vi "NIPKG Utility.vi"() -> ()   [LabVIEW 2017]
uses:
  <userlib>/_OpenG.lib/file/file.llb/Valid Path - Traditional__ogtk.vi
panel:
  out "State":string
  in  "Quit":bool
  in  "Tab Control":enum32{"Unpack NIPKG", "Pack NIPKG"}(tab)
  out "Unpack Complete?":bool
  out "Unpack Status":string
  in  "Unpack":bool
  in  "Path to .NIPKG":path
  in  "Unpack Destination":path
  in  "View Unpack Folder":bool
  in  "open":bool
  in  "Pack":bool
  in  "Path to Package Source":path
  in  "Pack Destination":path
  out "Pack Status":string
  in  "View Pack Folder":bool
  out "Pack Complete?":bool
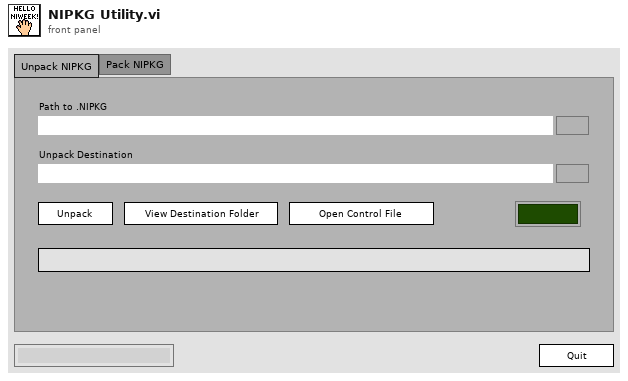
[diagram p1: front panel]
types:
  T1 = cluster{"unpack status":bool, "path to source":string, "pack destination":string, "pack status":string}
  T2 = cluster{"ready to unpack":bool, "path to nipkg":string, "unpack destination":string, "unpack status":string}
  T3 = cluster{"Core":cluster{"Current VI Reference":refnum<vi>, "Close Panel on Exit?":bool}, "unpack data":cluster{"ready to unpack":bool, "path to nipkg":string, "unpack destination":string, "unpack status":string}, "pack data":cluster{"ready to pack":bool, "path to source":string, "pack destination":string, "pack status":string}, "control path":string, "Unpack complete?":bool, "Pack complete?":bool}
  T4 = cluster{"ready to pack":bool, "path to source":string, "pack destination":string, "pack status":string}
  T5 = cluster{"Current VI Reference":refnum<vi>, "Close Panel on Exit?":bool}
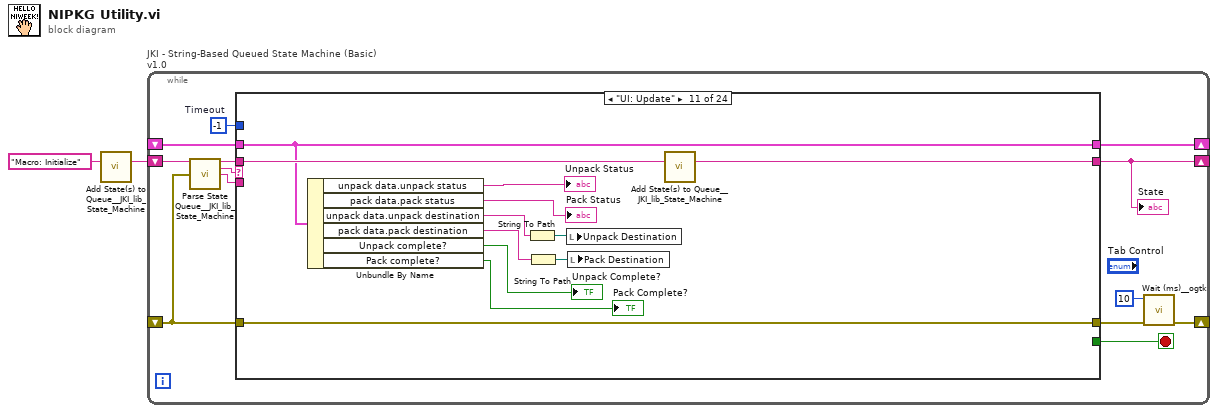
[diagram p0: block diagram]
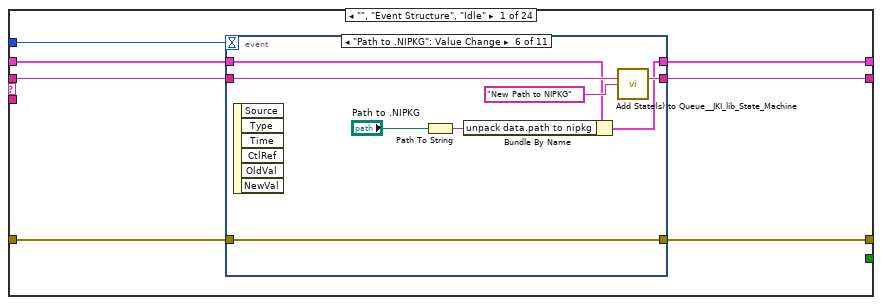
[diagram p2: hidden frame]
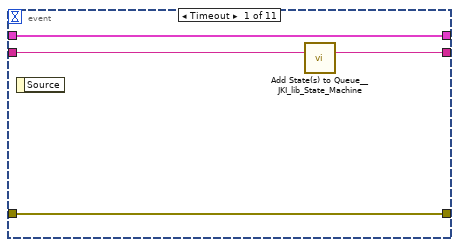
[diagram p3: hidden frame]
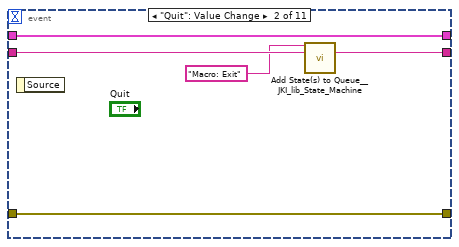
[diagram p4: hidden frame]
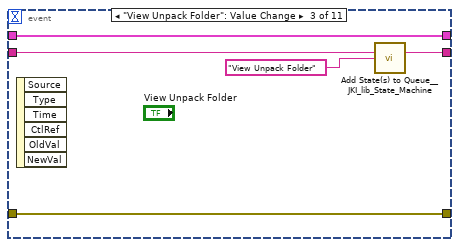
[diagram p5: hidden frame]
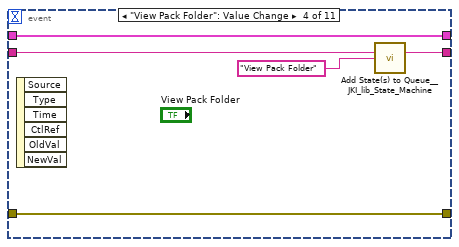
[diagram p6: hidden frame]
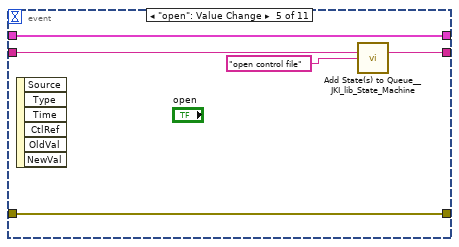
[diagram p7: hidden frame]
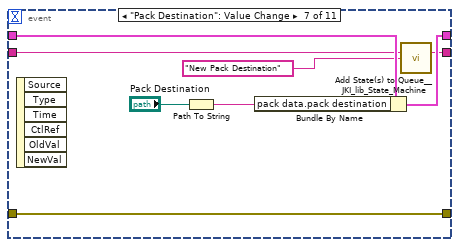
[diagram p8: hidden frame]
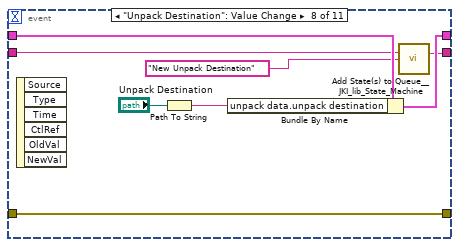
[diagram p9: hidden frame]
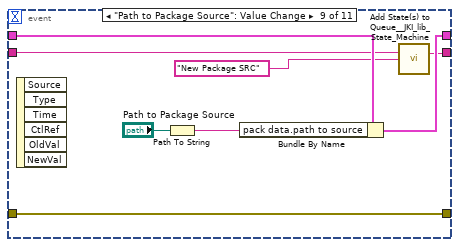
[diagram p10: hidden frame]
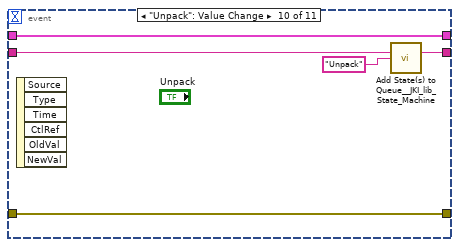
[diagram p11: hidden frame]
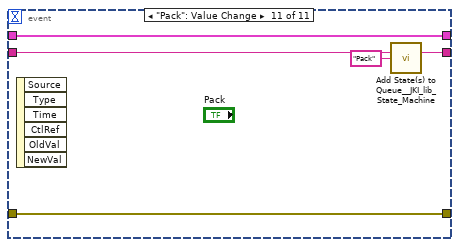
[diagram p12: hidden frame]
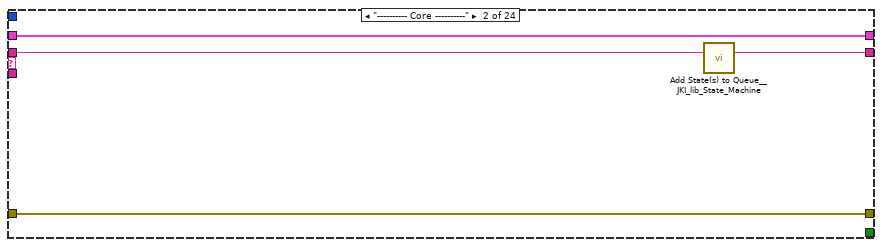
[diagram p13: hidden frame]
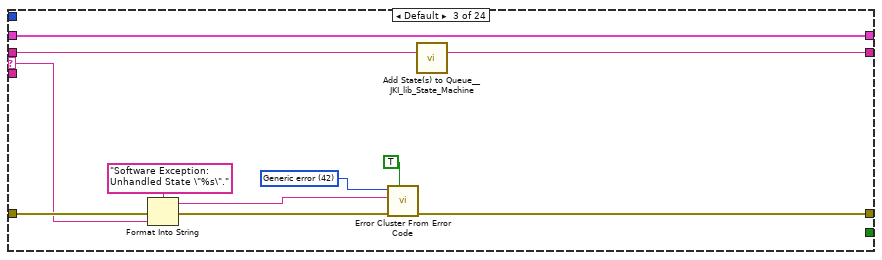
[diagram p14: hidden frame]
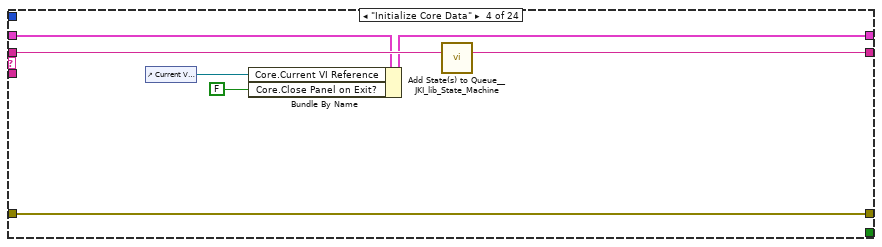
[diagram p15: hidden frame]
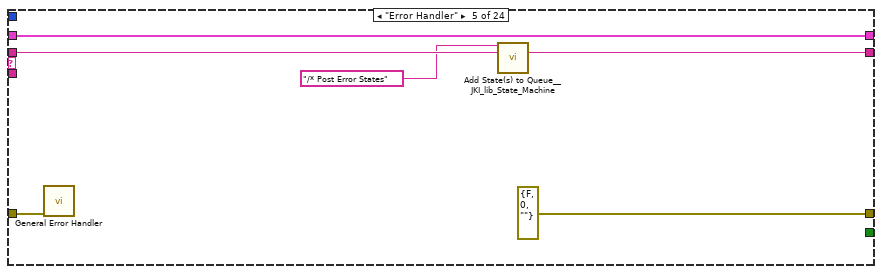
[diagram p16: hidden frame]
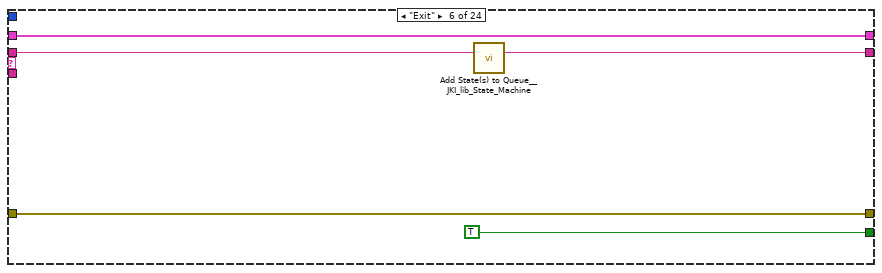
[diagram p17: hidden frame]
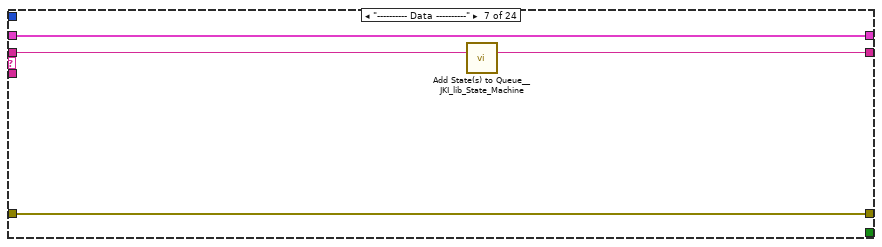
[diagram p18: hidden frame]
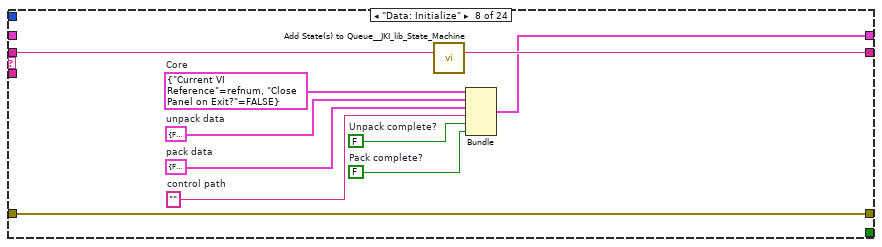
[diagram p19: hidden frame]
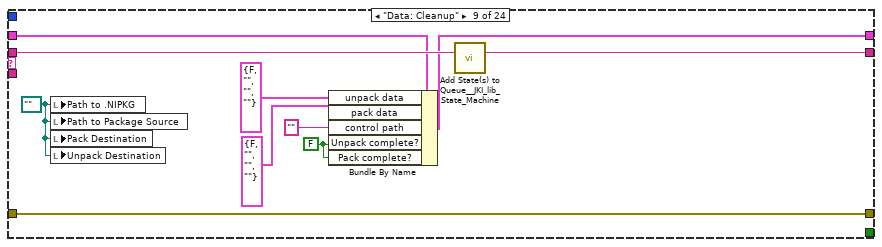
[diagram p20: hidden frame]
diagram:
  n1 = call <vilib>:"Add State(s) to Queue__JKI_lib_State_Machine.vi"("State(s) in (\"\")"="Macro: Initialize") -> ("States Out"=w1:string)  [unwired: 14 in]
  n2 = while "JKI - String-Based Queued State Machine (Basic) v1.0" {
    shift-right: [w10] -> _
    shift-left: _ -> [w9]
    shift-right: [w4] -> _
    shift-left: _ -> [w7]
    shift-right: [w6] -> _
    shift-left: w1 -> [w12]
    stop <- w11 stop-if-true
    w8 = -1  # Timeout
    n3 = call <vilib>:"Parse State Queue__JKI_lib_State_Machine.vi"("State Queue"=w12, "Error In (no error)"=w7) -> ("Remaining States"=w14:string, "Current State"=w15:string, "Arguments"=w13:string)  [unwired: 11 in]
    n4 = case shown="\"UI: Update\"" w15 {
      selector: w15 -> [_ _ w93 _ _ _ _ _ _ _ _ _ _ _ _ _ _ _ _ _ _ _ _ _]
      tunnel: w14 -> [w22 w92 w97 w110 w116 w121 w125 w135 w145 w149 w161 w165 w170 w177 w181 w198 w216 w224 w239 w256 w274 w296 w314 w329]
      tunnel: w13 -> [_ _ _ _ _ _ _ _ _ _ _ _ _ _ _ _ _ _ _ _ _ _ _ _]
      tunnel: w9 -> [w20 w89 w95 w106 w113 w119 w122 _ w142 w146 w158 w162 w167 w174 w178 w189 w207 w222 w237 w251 w269 w291 w309 w324]
      tunnel: [w19 w90 w99 w107 errorcluster {"status"=FALSE, "code"=0, "source"=""} ("error out") w118 w123 w132 w143 w147 w159 w163 w168 w175 w179 w195 w213 w220 w236 w253 w272 w294 w312 w327] -> w5
      tunnel: w7 -> [w18 w90 w98 w107 w112 w118 w123 w132 w143 w147 w159 w163 w168 w175 w179 w196 w214 w221 w235 w254 w272 w294 w312 w327]
      tunnel: [w21 w91 w96 w109 w115 w120 w124 w134 w144 w148 w160 w164 w169 w176 w180 w197 w215 w223 w238 w255 w273 w295 w313 w328] -> w6
      tunnel: [_ _ _ _ _ TRUE _ _ _ _ _ _ _ _ _ _ _ _ _ _ _ _ _ _] -> w11
      tunnel: [w17 w89 w95 w108 w113 w119 w122 w133 w141 w146 w158 w162 w167 w174 w178 w188 w206 w222 w237 w251 w270 w292 w310 w325] -> w10
      tunnel: w8 -> [w16 _ _ _ _ _ _ _ _ _ _ _ _ _ _ _ _ _ _ _ _ _ _ _]
      frame "", "Event Structure", "Idle" {
        n5 = event shown="[5] \"Path to .NIPKG\": Value Change" {
          selector: _ -> [_ _ _ _ _ _ _ _ _ _ _]
          dyn-events: _ -> [_ _ _ _ _ _ _ _ _ _ _]
          timeout: w16 -> [_ _ _ _ _ _ _ _ _ _ _]
          tunnel: w22 -> [w26 w31 w35 w40 w45 w53 w58 w66 w74 w82 w87]
          tunnel: [w25 w30 w36 w41 w46 w54 w60 w67 w75 w83 w88] -> w21
          tunnel: w20 -> [w23 w28 w34 w39 w42 w48 w61 w69 w77 w80 w85]
          tunnel: [w24 w29 w33 w38 w44 w51 w55 w63 w71 w81 w86] -> w19
          tunnel: w18 -> [w24 w29 w33 w38 w44 w51 w55 w63 w71 w81 w86]
          tunnel: [w23 w28 w34 w39 w42 w47 w62 w68 w76 w80 w85] -> w17
          event Timeout {
            n6 = event-data() -> ()  [unwired: 1 in, 1 out]
            n7 = call <vilib>:"Add State(s) to Queue__JKI_lib_State_Machine.vi"("State(s) in (\"\")"=w26) -> ("States Out"=w25:string)  [unwired: 14 in]
          }
          event "Quit": Value Change {
            n8 = event-data() -> ()  [unwired: 1 in, 1 out]
            n9 = call <vilib>:"Add State(s) to Queue__JKI_lib_State_Machine.vi"("State(s) in Front (\"\")"="Macro: Exit", "State(s) in (\"\")"=w31) -> ("States Out"=w30:string)  [unwired: 13 in]
          }
          event "View Unpack Folder": Value Change {
            n10 = event-data() -> ()  [unwired: 1 in, 6 out]
            n11 = call <vilib>:"Add State(s) to Queue__JKI_lib_State_Machine.vi"("State(s) in (\"\")"=w35, "State(s) at Back (\"\")"="View Unpack Folder" ("State(s) at Back (\"\")")) -> ("States Out"=w36:string)  [unwired: 13 in]
          }
          event "View Pack Folder": Value Change {
            n12 = event-data() -> ()  [unwired: 1 in, 6 out]
            n13 = call <vilib>:"Add State(s) to Queue__JKI_lib_State_Machine.vi"("State(s) in (\"\")"=w40, "State(s) at Back (\"\")"="View Pack Folder" ("State(s) at Back (\"\")")) -> ("States Out"=w41:string)  [unwired: 13 in]
          }
          event "open": Value Change {
            n14 = event-data() -> ()  [unwired: 1 in, 6 out]
            n15 = call <vilib>:"Add State(s) to Queue__JKI_lib_State_Machine.vi"("State(s) in (\"\")"=w45, "State(s) at Back (\"\")"="open control file") -> ("States Out"=w46:string)  [unwired: 13 in]
          }
          event "Path to .NIPKG": Value Change {
            n16 = event-data() -> ()  [unwired: 1 in, 6 out]
            n17 = Path To String(path="Path to .NIPKG") -> (string=w49:string)
            n18 = Bundle By Name(cluster=w48, "unpack data.path to nipkg"=w49) -> (w47:T3)
            n19 = call <vilib>:"Add State(s) to Queue__JKI_lib_State_Machine.vi"("State(s) in (\"\")"=w53, "State(s) at Back (\"\")"="New Path to NIPKG" ("State(s) at Back (\"\")")) -> ("States Out"=w54:string)  [unwired: 13 in]
          }
          event "Pack Destination": Value Change {
            n20 = event-data() -> ()  [unwired: 1 in, 6 out]
            n21 = Path To String(path="Pack Destination") -> (string=w59:string)
            n22 = Bundle By Name(cluster=w61, "pack data.pack destination"=w59) -> (w62:T3)
            n23 = call <vilib>:"Add State(s) to Queue__JKI_lib_State_Machine.vi"("State(s) in (\"\")"=w58, "State(s) at Back (\"\")"="New Pack Destination" ("State(s) at Back (\"\")")) -> ("States Out"=w60:string)  [unwired: 13 in]
          }
          event "Unpack Destination": Value Change {
            n24 = event-data() -> ()  [unwired: 1 in, 6 out]
            n25 = Path To String(path="Unpack Destination") -> (string=w70:string)
            n26 = Bundle By Name(cluster=w69, "unpack data.unpack destination"=w70) -> (w68:T3)
            n27 = call <vilib>:"Add State(s) to Queue__JKI_lib_State_Machine.vi"("State(s) in (\"\")"=w66, "State(s) at Back (\"\")"="New Unpack Destination" ("State(s) at Back (\"\")")) -> ("States Out"=w67:string)  [unwired: 13 in]
          }
          event "Path to Package Source": Value Change {
            n28 = event-data() -> ()  [unwired: 1 in, 6 out]
            n29 = Path To String(path="Path to Package Source") -> (string=w78:string)
            n30 = Bundle By Name(cluster=w77, "pack data.path to source"=w78) -> (w76:T3)
            n31 = call <vilib>:"Add State(s) to Queue__JKI_lib_State_Machine.vi"("State(s) in (\"\")"=w74, "State(s) at Back (\"\")"="New Package SRC" ("State(s) at Back (\"\")")) -> ("States Out"=w75:string)  [unwired: 13 in]
          }
          event "Unpack": Value Change {
            n32 = event-data() -> ()  [unwired: 1 in, 6 out]
            n33 = call <vilib>:"Add State(s) to Queue__JKI_lib_State_Machine.vi"("State(s) in (\"\")"=w82, "State(s) at Back (\"\")"="Unpack" ("State(s) at Back (\"\")")) -> ("States Out"=w83:string)  [unwired: 13 in]
          }
          event "Pack": Value Change {
            n34 = event-data() -> ()  [unwired: 1 in, 6 out]
            n35 = call <vilib>:"Add State(s) to Queue__JKI_lib_State_Machine.vi"("State(s) in (\"\")"=w87, "State(s) at Back (\"\")"="Pack" ("State(s) at Back (\"\")")) -> ("States Out"=w88:string)  [unwired: 13 in]
          }
        }
      }
      frame "---------- Core ----------" {
        n36 = call <vilib>:"Add State(s) to Queue__JKI_lib_State_Machine.vi"("State(s) in (\"\")"=w92) -> ("States Out"=w91:string)  [unwired: 14 in]
      }
      frame Default {
        w102 = 42 items=["No error", "Argument error", "Memory is full", "Out of zone", "End of file", "File already open", "Generic file I/O error", "File not found", "File permission error", "Disk is full", "Duplicate path", "Too many files open", "System feature not enabled", "Resource file not found", "Cannot add resource", "Resource not found", "Image not found", "Image memory error", "Pen does not exist", "Config type invalid", "Config token not found", "Config parse error", "Config memory error", "Bad external code format", "Bad external code offset", "External code not present", "Null window", "Destroy window error", "Null menu", "Print aborted", "Bad print record", "Print driver error", "Windows error during printing", "Memory error during printing", "Print dialog error", "Generic print error", "Invalid device refnum", "Device not found", "Device parameter error", "Device unit error", "Cannot open device", "Device call aborted", "Generic error", "Cancelled by user", "Object ID too low", "Object ID too high", "Object not in heap", "Unknown heap", "Unknown object (invalid DefProc)", "Unknown object (DefProc not in table)", "Message out of range", "Invalid (null) method", "Unknown message", "Manager call not supported", "Bad address", "Network operation in progress", "Network operation timed out", "Connection is busy", "Network attribute not supported", "Network error", "Address in use", "System out of memory", "Connection aborted", "Connection refused", "Not connected", "Already connected", "Connection closed", "Initialization error (interapplication manager)", "Bad occurrence", "Wait on unbound occurrence handler", "Occurrence queue overflow", "Datalog type conflict", "Unused", "Unrecognized type (interapplication manager)", "Memory corrupt", "Failed to make temporary DLL", "Old CIN version", "Drag socket not found", "Failed to load drop-object", "Failed to register OLE object", "Failed to release OLE object", "Format specifier type mismatch", "Unknown format specifier", "Too few format specifiers", "Too many format specifiers", "Scan failed", "Newer CIN version", "Error converting to variant", "Runtime menu error", "Password tampered", "Variant attribute not found", "Incompatible variant data type", "Event data is not available", "Event Store is not present", "Occurrence is not found", "Event Queue is not created", "Event info is not available", "Refnum passed is NULL", "Error retrieving Class GUID", "Error retrieving CoClass GUID", "Error retrieving TypeLib GUID.", "Bad built application magic bytes.", "Specific driver is different from the specific driver associated with the Logical Name.", "There is no session opened to the class driver.", "Max Error", "MAX - Error with config objects", "MAX - Error loading configuration", "MAX - Group not supported"]
        n37 = Format Into String(format string="Software Exception: Unhandled State \"%s\"." ("message"), error in=w98, w93) -> (resulting string=w101:string, error out=w100:errorcluster)  [unwired: 1 in]
        n38 = call <vilib>:"Error Cluster From Error Code.vi"("show call chain? (False)"=TRUE, "error in (no error)"=w100, "error message (\"\")"=w101, "error code (0)"=w102) -> ("error out"=w99:errorcluster)  [unwired: 5 in]
        n39 = call <vilib>:"Add State(s) to Queue__JKI_lib_State_Machine.vi"("State(s) in (\"\")"=w97) -> ("States Out"=w96:string)  [unwired: 14 in]
      }
      frame "Initialize Core Data" {
        n40 = control-ref of="Current VI Reference"() -> (w105:refnum<vi>)
        n41 = Bundle By Name(cluster=w106, "Core.Current VI Reference"=w105, "Core.Close Panel on Exit?"=FALSE) -> (w108:T3)
        n42 = call <vilib>:"Add State(s) to Queue__JKI_lib_State_Machine.vi"("State(s) in (\"\")"=w110) -> ("States Out"=w109:string)  [unwired: 14 in]
      }
      frame "Error Handler" {
        n43 = call <vilib>:"General Error Handler.vi"("error in (no error)"=w112) -> ()  [unwired: 10 in, 5 out]
        n44 = call <vilib>:"Add State(s) to Queue__JKI_lib_State_Machine.vi"("State(s) in Front (\"\")"="/* Post Error States", "State(s) in (\"\")"=w116) -> ("States Out"=w115:string)  [unwired: 13 in]
      }
      frame "Exit" {
        n45 = call <vilib>:"Add State(s) to Queue__JKI_lib_State_Machine.vi"("State(s) in (\"\")"=w121) -> ("States Out"=w120:string)  [unwired: 14 in]
      }
      frame "---------- Data ----------" {
        n46 = call <vilib>:"Add State(s) to Queue__JKI_lib_State_Machine.vi"("State(s) in (\"\")"=w125) -> ("States Out"=w124:string)  [unwired: 14 in]
      }
      frame "Data: Initialize" {
        w126 = FALSE  # Pack complete?
        w127 = FALSE  # Unpack complete?
        w128 = ""  # control path
        w129 = T4 {"ready to pack"=FALSE, "path to source"="", "pack destination"="", "pack status"="Please specify the path to the ni package source folder..."}  # pack data
        w130 = T2 {"ready to unpack"=FALSE, "path to nipkg"="", "unpack destination"="", "unpack status"="Please specify the path to an NI package file..."}  # unpack data
        w131 = T5 {"Current VI Reference"=refnum, "Close Panel on Exit?"=FALSE}  # Core
        n47 = call <vilib>:"Add State(s) to Queue__JKI_lib_State_Machine.vi"("State(s) in (\"\")"=w135) -> ("States Out"=w134:string)  [unwired: 14 in]
        n48 = Bundle("Core"=w131, "unpack data"=w130, "pack data"=w129, "control path"=w128, "Unpack complete?"=w127, "Pack complete?"=w126) -> (w133:T3)  [unwired: 1 in]
      }
      frame "Data: Cleanup" {
        w136 = FALSE
        w137 = path "" ("Path to .NIPKG")
        n49 = local write "Path to .NIPKG"(w137) -> ()
        n50 = local write "Path to Package Source"(w137) -> ()
        n51 = local write "Pack Destination"(w137) -> ()
        n52 = local write "Unpack Destination"(w137) -> ()
        n53 = Bundle By Name(cluster=w142, "unpack data"=T2 {"ready to unpack"=FALSE, "path to nipkg"="", "unpack destination"="", "unpack status"=""}, "pack data"=T1 {"unpack status"=FALSE, "path to source"="", "pack destination"="", "pack status"=""}, "control path"="", "Unpack complete?"=w136, "Pack complete?"=w136) -> (w141:T3)
        n54 = call <vilib>:"Add State(s) to Queue__JKI_lib_State_Machine.vi"("State(s) in (\"\")"=w145) -> ("States Out"=w144:string)  [unwired: 14 in]
      }
      frame "---------- UI ----------" {
        n55 = call <vilib>:"Add State(s) to Queue__JKI_lib_State_Machine.vi"("State(s) in (\"\")"=w149) -> ("States Out"=w148:string)  [unwired: 14 in]
      }
      frame "UI: Update" {
        n56 = Unbundle By Name(w158) -> ("unpack data.unpack status"=→"Unpack Status":string, "pack data.pack status"=→"Pack Status":string, "unpack data.unpack destination"=w153:string, "pack data.pack destination"=w152:string, "Unpack complete?"=→"Unpack Complete?":bool, "Pack complete?"=→"Pack Complete?":bool)
        n57 = String To Path(string=w153) -> (path=w155:path)
        n58 = String To Path(string=w152) -> (path=w154:path)
        n59 = local write "Unpack Destination"(w155) -> ()
        n60 = local write "Pack Destination"(w154) -> ()
        n61 = call <vilib>:"Add State(s) to Queue__JKI_lib_State_Machine.vi"("State(s) in (\"\")"=w161) -> ("States Out"=w160:string)  [unwired: 14 in]
      }
      frame "---------- Macro ----------" {
        n62 = call <vilib>:"Add State(s) to Queue__JKI_lib_State_Machine.vi"("State(s) in (\"\")"=w165) -> ("States Out"=w164:string)  [unwired: 14 in]
      }
      frame "Macro: Initialize" {
        n63 = call <vilib>:"Add State(s) to Queue__JKI_lib_State_Machine.vi"("State(s) in Front (\"\")"="Data: Initialize\nInitialize Core Data\nUI: Update", "State(s) in (\"\")"=w170) -> ("States Out"=w169:string)  [unwired: 13 in]
      }
      frame "Macro: Exit" {
        n64 = call <vilib>:"Add State(s) to Queue__JKI_lib_State_Machine.vi"("State(s) in (\"\")"="", "State(s) at Back (\"\")"="Data: Cleanup\nUI: Update\nExit") -> ("States Out"=w172:string)  [unwired: 13 in]
        n65 = call <vilib>:"Add State(s) to Queue__JKI_lib_State_Machine.vi"("State(s) in Front (\"\")"=w172, "State(s) in (\"\")"=w177) -> ("States Out"=w176:string)  [unwired: 13 in]
      }
      frame "---------- New Category ----------" {
        n66 = call <vilib>:"Add State(s) to Queue__JKI_lib_State_Machine.vi"("State(s) in (\"\")"=w181) -> ("States Out"=w180:string)  [unwired: 14 in]
      }
      frame "Unpack" {
        w190 = "\""
        n67 = Unbundle By Name(w189) -> ("unpack data.path to nipkg"=w192:string, "unpack data.unpack destination"=w191:string)
        n68 = call <vilib>:"Space Constant.vi"() -> ("String"=w186:string)
        n69 = Concatenate Strings("cmd /c nipkg.exe", w186, "unpack", w186, w190, w192, w190, w186, w190, w191, w190) -> (w184:string)
        n70 = call <vilib>:"Add State(s) to Queue__JKI_lib_State_Machine.vi"("State(s) in (\"\")"=w198, "State(s) at Back (\"\")"="View Unpack Folder\nUI: Update" ("State(s) at Back (\"\")")) -> ("States Out"=w197:string)  [unwired: 13 in]
        n71 = call <vilib>:"System Exec.vi"("error in (no error)"=w196, "working directory"=path "c:/program files/national instruments/ni package manager", "command line"=w184) -> ("error out"=w195:errorcluster)  [unwired: 5 in, 3 out]
        n72 = Bundle By Name(cluster=w189, "unpack data.unpack status"="Unpacking complete!" ("string"), "Unpack complete?"=TRUE) -> (w188:T3)
      }
      frame "Pack" {
        w208 = "\""
        n73 = Unbundle By Name(w207) -> ("pack data.path to source"=w210:string, "pack data.pack destination"=w209:string)
        n74 = call <vilib>:"Space Constant.vi"() -> ("String"=w204:string)
        n75 = Concatenate Strings("cmd /c nipkg.exe", w204, "pack", w204, w208, w210, w208, w204, w208, w209, w208) -> (w202:string)
        n76 = call <vilib>:"Add State(s) to Queue__JKI_lib_State_Machine.vi"("State(s) in (\"\")"=w216, "State(s) at Back (\"\")"="View Pack Folder\nUI: Update" ("State(s) at Back (\"\")")) -> ("States Out"=w215:string)  [unwired: 13 in]
        n77 = call <vilib>:"System Exec.vi"("error in (no error)"=w214, "working directory"=path "c:/program files/national instruments/ni package manager", "command line"=w202) -> ("error out"=w213:errorcluster)  [unwired: 5 in, 3 out]
        n78 = Bundle By Name(cluster=w207, "pack data.pack status"="Packing complete!" ("string"), "pack data.ready to pack"=FALSE, "Pack complete?"=TRUE) -> (w206:T3)
      }
      frame "View Unpack Folder" {
        n79 = Unbundle By Name(w222) -> ("unpack data.unpack destination"=w218:string)
        n80 = String To Path(string=w218) -> (path=w219:path)
        n81 = call-poly <userlib>:"Valid Path__ogtk.vi"("path"=w219) -> ("valid"=w217:bool)
        n82 = case shown="True" w217 {
          tunnel: w221 -> [w225 w231]
          tunnel: [w225 w230] -> w220
          tunnel: w218 -> [_ w226]
          frame False {
          }
          frame True {
            n83 = Concatenate Strings("explorer.exe /select,\"", w226, "\"" ("string")) -> (w227:string)
            n84 = call <vilib>:"System Exec.vi"("error in (no error)"=w231, "command line"=w227) -> ("error out"=w230:errorcluster)  [unwired: 6 in, 3 out]
          }
        }
        n85 = call <vilib>:"Add State(s) to Queue__JKI_lib_State_Machine.vi"("State(s) in (\"\")"=w224) -> ("States Out"=w223:string)  [unwired: 14 in]
      }
      frame "View Pack Folder" {
        n86 = Unbundle By Name(w237) -> ("pack data.pack destination"=w233:string)
        n87 = String To Path(string=w233) -> (path=w234:path)
        n88 = call-poly <userlib>:"Valid Path__ogtk.vi"("path"=w234) -> ("valid"=w232:bool)
        n89 = case shown="True" w232 {
          tunnel: [w240 w243] -> w236
          tunnel: w235 -> [w240 w242]
          tunnel: w233 -> [_ w241]
          frame False {
          }
          frame True {
            n90 = Concatenate Strings("explorer.exe /select,\"", w241, "\"" ("string")) -> (w244:string)
            n91 = call <vilib>:"System Exec.vi"("error in (no error)"=w242, "command line"=w244) -> ("error out"=w243:errorcluster)  [unwired: 6 in, 3 out]
          }
        }
        n92 = call <vilib>:"Add State(s) to Queue__JKI_lib_State_Machine.vi"("State(s) in (\"\")"=w239) -> ("States Out"=w238:string)  [unwired: 14 in]
      }
      frame "open control file" {
        n93 = Unbundle By Name(w251) -> ("unpack data.unpack destination"=w250:string)
        n94 = Concatenate Strings(w250, "\\control" ("string")) -> (w249:string)
        n95 = String To Path(string=w249) -> (path=w248:path)
        n96 = call-poly <userlib>:"Valid Path__ogtk.vi"("path"=w248) -> ("valid"=w247:bool)
        n97 = case shown="True" w247 {
          tunnel: w254 -> [w257 w261]
          tunnel: [w257 w260] -> w253
          tunnel: w248 -> [_ w258]
          frame False {
          }
          frame True {
            n98 = call <vilib>:"System Exec.vi"("error in (no error)"=w261, "working directory"=w258, "command line"="cmd /c start notepad control") -> ("error out"=w260:errorcluster)  [unwired: 5 in, 3 out]
          }
        }
        n99 = call <vilib>:"Add State(s) to Queue__JKI_lib_State_Machine.vi"("State(s) in (\"\")"=w256) -> ("States Out"=w255:string)  [unwired: 14 in]
      }
      frame "New Path to NIPKG" {
        n100 = Unbundle By Name(w269) -> ("unpack data.path to nipkg"=w267:string)
        n101 = String To Path(string=w267) -> (path=w266:path)
        n102 = call-poly <userlib>:"Valid Path__ogtk.vi"("path"=w266) -> ("valid"=w268:bool)
        n103 = case shown="True" w268 {
          tunnel: w266 -> [_ w283]
          tunnel: [path "" ("appended path") w280] -> w265
          tunnel: [FALSE TRUE] -> w263
          tunnel: ["Please enter a valid path to the package file..." ("f") "Ready to unpack..." ("t")] -> w262
          frame False {
          }
          frame True {
            n104 = Strip Path(path=w283) -> (stripped path=w282:path)  [unwired: 1 out]
            n105 = Build Path(base path=w282, name or relative path="pkgsrc") -> (appended path=w280:path)
          }
        }
        n106 = Path To String(path=w265) -> (string=w264:string)
        n107 = Bundle By Name(cluster=w269, "unpack data.unpack destination"=w264, "unpack data.ready to unpack"=w263, "unpack data.unpack status"=w262) -> (w270:T3)
        n108 = call <vilib>:"Add State(s) to Queue__JKI_lib_State_Machine.vi"("State(s) in (\"\")"=w274, "State(s) at Back (\"\")"="UI: Update" ("State(s) at Back (\"\")")) -> ("States Out"=w273:string)  [unwired: 13 in]
      }
      frame "New Package SRC" {
        n109 = Unbundle By Name(w291) -> ("pack data.path to source"=w289:string)
        n110 = String To Path(string=w289) -> (path=w288:path)
        n111 = call-poly <userlib>:"Valid Path__ogtk.vi"("path"=w288) -> ("valid"=w290:bool)
        n112 = case shown="False" w290 {
          tunnel: w288 -> [_ w303]
          tunnel: [path "" ("appended path") w300] -> w287
          tunnel: [FALSE TRUE] -> w285
          tunnel: ["Please enter a valid path to the source..." ("f") "Ready to pack..." ("t")] -> w284
          frame False {
          }
          frame True {
            n113 = Strip Path(path=w303) -> (stripped path=w300:path)  [unwired: 1 out]
          }
        }
        n114 = Path To String(path=w287) -> (string=w286:string)
        n115 = Bundle By Name(cluster=w291, "pack data.pack destination"=w286, "pack data.ready to pack"=w285, "pack data.pack status"=w284) -> (w292:T3)
        n116 = call <vilib>:"Add State(s) to Queue__JKI_lib_State_Machine.vi"("State(s) in (\"\")"=w296, "State(s) at Back (\"\")"="UI: Update" ("State(s) at Back (\"\")")) -> ("States Out"=w295:string)  [unwired: 13 in]
      }
      frame "New Pack Destination" {
        n117 = Unbundle By Name(w309) -> ("pack data.pack destination"=w304:string)
        n118 = String To Path(string=w304) -> (path=w307:path)
        n119 = call-poly <userlib>:"Valid Path__ogtk.vi"("path"=w307) -> ("valid"=w308:bool)
        n120 = case shown="False" w308 {
          tunnel: [FALSE TRUE] -> w306
          tunnel: ["Please enter a valid destination path..." ("f") "Ready to unpack..." ("t")] -> w305
          frame False {
          }
          frame True {
          }
        }
        n121 = Bundle By Name(cluster=w309, "pack data.ready to pack"=w306, "pack data.pack destination"=w305) -> (w310:T3)
        n122 = call <vilib>:"Add State(s) to Queue__JKI_lib_State_Machine.vi"("State(s) in (\"\")"=w314, "State(s) at Back (\"\")"="UI: Update" ("State(s) at Back (\"\")")) -> ("States Out"=w313:string)  [unwired: 13 in]
      }
      frame "New Unpack Destination" {
        n123 = Unbundle By Name(w324) -> ("unpack data.unpack destination"=w319:string)
        n124 = String To Path(string=w319) -> (path=w322:path)
        n125 = call-poly <userlib>:"Valid Path__ogtk.vi"("path"=w322) -> ("valid"=w323:bool)
        n126 = case shown="False" w323 {
          tunnel: [FALSE TRUE] -> w321
          tunnel: ["Please enter a valid destination path..." ("f") "Ready to unpack..." ("t")] -> w320
          frame False {
          }
          frame True {
          }
        }
        n127 = Bundle By Name(cluster=w324, "unpack data.ready to unpack"=w321, "unpack data.unpack status"=w320) -> (w325:T3)
        n128 = call <vilib>:"Add State(s) to Queue__JKI_lib_State_Machine.vi"("State(s) in (\"\")"=w329, "State(s) at Back (\"\")"="UI: Update" ("State(s) at Back (\"\")")) -> ("States Out"=w328:string)  [unwired: 13 in]
      }
    }
    "State" <- w6
    n129 = call <userlib>:"Wait (ms)__ogtk.vi"("error in (no error)"=w5, "milliseconds to wait"=u32 10) -> ("error out"=w4:errorcluster)  [unwired: 8 in, 1 out]
  }
